vi "integrator_limited.vi"(1 "Lower_Limit":dbl, 2 "Upper_Limit":dbl, 3 "Dt":dbl, 4 "Ic":bool, 5 "Ic_value":dbl, 6 "In":dbl) -> (0 "Out":dbl)   [LabVIEW 2023]
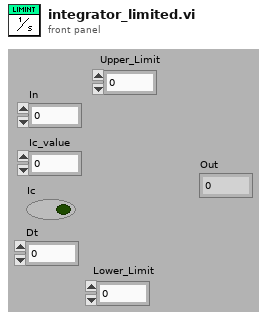
[diagram p1: front panel]
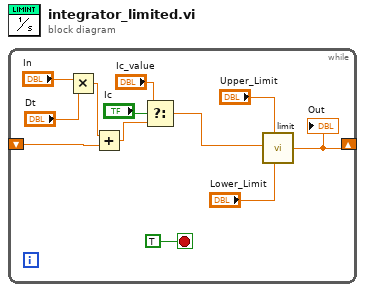
[diagram p0: block diagram]
diagram:
  n1 = while {
    shift-right: [w1] -> _
    shift-left: _ -> [w11]
    stop <- TRUE stop-if-true
    n2 = Multiply(x="In", y="Dt") -> (x*y=w8:dbl)
    n3 = Add(x=w8, y=w11) -> (x+y=w5:dbl)
    n4 = Select(t="Ic_value", s="Ic", f=w5) -> (s? t:f=w4:dbl)
    n5 = call "limit.vi"("Lower_Limit"="Lower_Limit", "Upper_Limit"="Upper_Limit", "Input"=w4) -> ("Output"=w1:dbl)  [unwired: 3 in]
    "Out" <- w1
  }
